vi "Osc_SinWave.vi"(1 "Reset":bool, 2 "WaveType":enum16{"sin", "cos"}(ring), 3 "Phase":dbl format="%#_13g", 4 "step_t":dbl format="%#_13g", 5 "Frequency/Hz":dbl format="%#_13g", 6 "Amplitude":dbl format="%#_13g") -> (0 "Wave":dbl(graph))   [LabVIEW 2014]
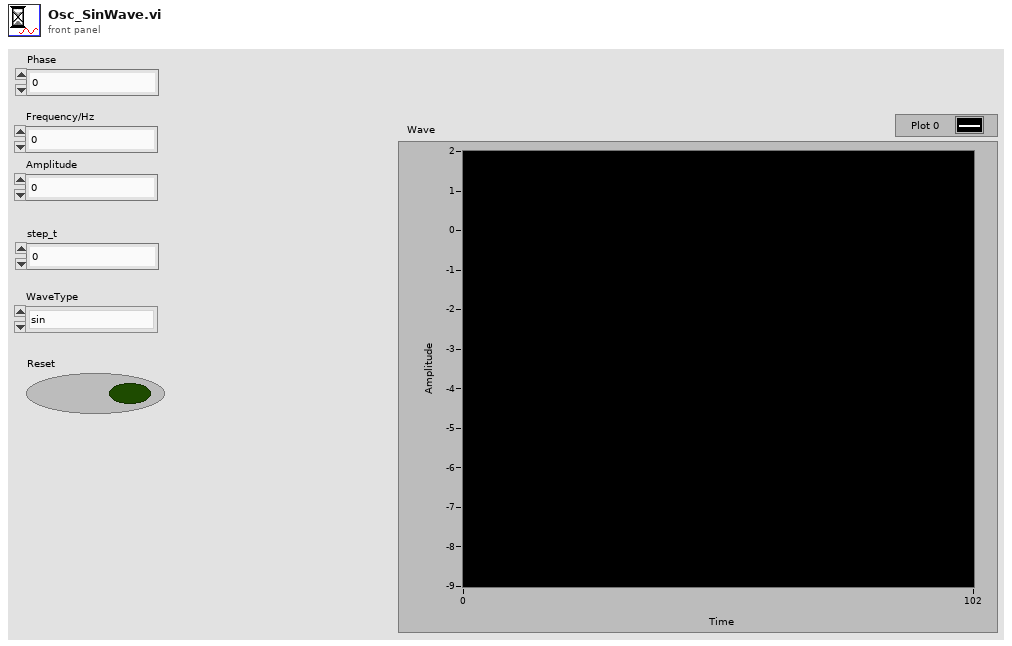
[diagram p1: front panel]
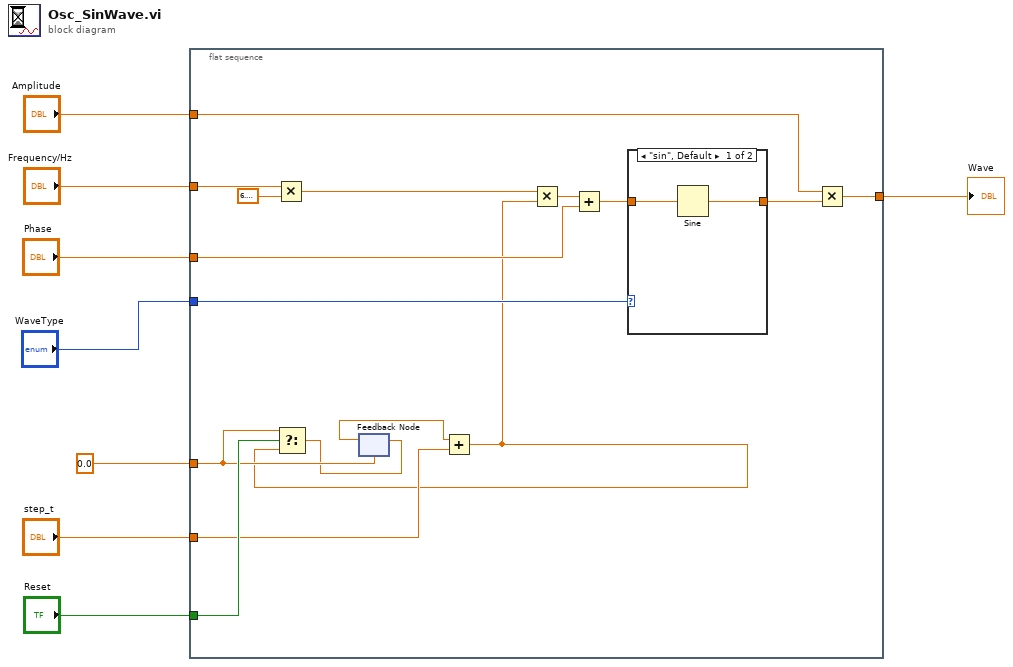
[diagram p0: block diagram]
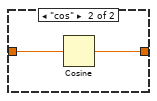
[diagram p2: hidden frame]
diagram:
  n1 = flat-sequence {
    tunnel: "Amplitude" -> [w9]
    tunnel: "Frequency/Hz" -> [w24]
    tunnel: 0.0 ("Init_t_bias") -> [w21]
    tunnel: "Phase" -> [w17]
    tunnel: "step_t" -> [w13]
    tunnel: "Reset" -> [w22]
    tunnel: "WaveType" -> [w15]
    tunnel: [w10] -> w2
    frame #0 {
      n2 = Multiply(x=w24, y=6.283185307179586) -> (x*y=w19:dbl)
      n3 = feedback #1(w21) -> (w14:dbl)
      n4 = Add(x=w14, y=w13) -> (x+y=w12:dbl)
      n5 = Select(t=w21, s=w22, f=w12) -> (s? t:f=w20:dbl)
      n6 = feedback-in #1(w20) -> ()
      n7 = Multiply(x=w19, y=w12) -> (x*y=w18:dbl)
      n8 = Add(x=w18, y=w17) -> (x+y=w16:dbl)
      n9 = case shown="\"sin\", Default" w15 {
        tunnel: w16 -> [w26 w28]
        tunnel: [w25 w27] -> w11
        frame "sin", Default {
          n10 = Sine(x=w26) -> (sin(x)=w25:dbl)
        }
        frame "cos" {
          n11 = Cosine(x=w28) -> (cos(x)=w27:dbl)
        }
      }
      n12 = Multiply(x=w9, y=w11) -> (x*y=w10:dbl)
    }
  }
  "Wave" <- w2
